vi "Convert Hz to mel.vi"(11 "Hz":dbl) -> (3 "mel":dbl)   [LabVIEW 2011]
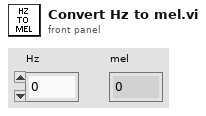
[diagram p1: front panel]
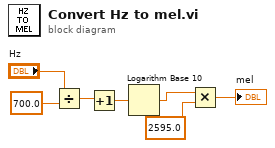
[diagram p0: block diagram]
diagram:
  n1 = Divide(x="Hz", y=700.0) -> (x/y=w3:dbl)
  n2 = Increment(x=w3) -> (x+1=w4:dbl)
  n3 = Logarithm Base 10(1:w4) -> (0:w5:dbl)
  n4 = Multiply(x=w5, y=2595.0) -> (x*y=→"mel":dbl)
